vi "FindhInPlane.vi"(3 "Full h(r,t)":bool, 4 "Variables in":T1={"Number of rings"=1, "sound spd (cm/s)"=150000, "z span (cm)"=4.0, "z steps"=20, "y span (cm)"=50.0, "y steps"=0, "time step (s)"=1e-08, "z"=0.0, "y"=0.0, "ref delay"=0.0, "freq (MHz)"=4.71, "cycles"=300} {"freq (MHz)" format="%.2f"; "z span (cm)" format="%.2f"; "y" format="%.2f"; "ref delay" format="%.2f"; "y span (cm)" format="%.2f"; "z" format="%.2f"; "time step (s)" format="%.2e"}, 5 "Trans Geometry":cluster{"Radius":dbl, "a":dbl}={"Radius"=4.8, "a"=1.0} {"a" format="%.2f"; "Radius" format="%.2f"}) -> (0 "Y axis":dbl[](array[numeric]) format="%.2f", 1 "h(r,t)":dbl[][](array[numeric]) format="%.2f", 2 "delay pts":i32[](array[numeric]))   [LabVIEW 2022 SP3]
uses:
  <vilib>/Math Plots/3D Math Plots/3D Surface/3D Surface XCtrl/3D Surface.xctl
  <vilib>/Math Plots/3D Math Plots/3D Surface/3D Surface Datatype/Public/Plot Helper (Matrix).vi
  <vilib>/Math Plots/3D Math Plots/3D Surface/3D Surface Datatype/3D Surface Datatype.lvclass
panel:
  out "3D Surface":refnum<class "3D Plot Datatype.lvclass">[](xcontrol)
  in  "Display 3-D?":bool
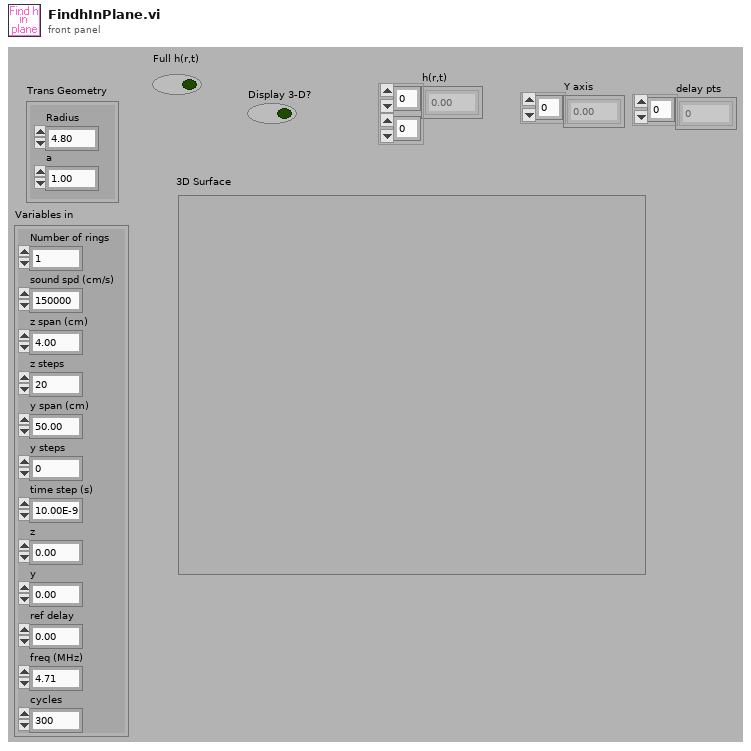
[diagram p1: front panel]
types:
  T1 = cluster{"Number of rings":i32, "sound spd (cm/s)":i32, "z span (cm)":dbl, "z steps":i32, "y span (cm)":dbl, "y steps":i32, "time step (s)":sgl, "z":dbl, "y":dbl, "ref delay":dbl, "freq (MHz)":dbl, "cycles":i32}
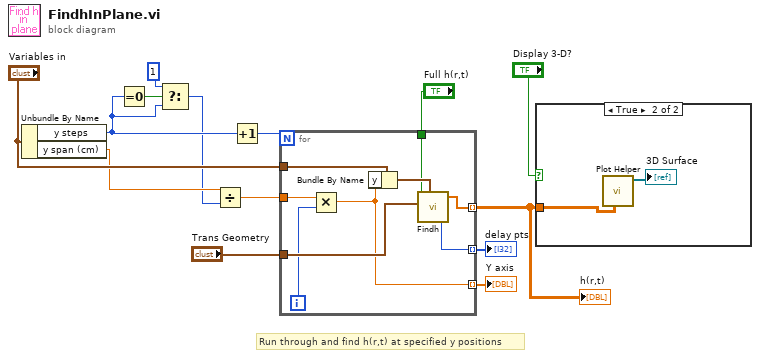
[diagram p0: block diagram]
diagram:
  # "Run through and find h(r,t) at specified y positions"
  n1 = Unbundle By Name("Variables in") -> ("y steps"=w3:i32, "y span (cm)"=w9:dbl)
  n2 = Equal To 0?(x=w3) -> (x = 0?=w4:bool)
  n3 = Select(t=1, s=w4, f=w3) -> (s? t:f=w2:i32)
  n4 = Divide(x=w9, y=w2) -> (x/y=w8:dbl)
  n5 = Increment(x=w3) -> (x+1=w7:i32)
  n6 = for {
    N: w7 -> [_]
    tunnel: "Trans Geometry" -> [w23]
    tunnel: w8 -> [w21]
    tunnel: [w20] -> w14 mode=indexing
    tunnel: "Variables in" -> [w19]
    tunnel: [w18] -> w12 mode=indexing
    tunnel: [w16] -> w6 mode=indexing
    tunnel: "Full h(r,t)" -> [w15]
    i -> [w22]
    n7 = Multiply(x=w21, y=w22) -> (x*y=w18:dbl)
    n8 = Bundle By Name(cluster=w19, "y"=w18) -> (w17:T1)
    n9 = call "Findh.vi"("Full h(r,t)"=w15, "Trans Geometry"=w23, "Variables in"=w17) -> ("h(r,t)"=w20:dbl[], "delay pts"=w16:i32)  [unwired: 3 out]
  }
  "h(r,t)" <- w14
  "Y axis" <- w12
  "delay pts" <- w6
  n10 = case shown="True" "Display 3-D?" {
    tunnel: w14 -> [_ w24]
    frame False {
    }
    frame True {
      n11 = call-poly <vilib>:"Plot Helper.vi"("z matrix"=w24) -> ("3D Plot lvclass Array out"=→"3D Surface":refnum<class "3D Plot Datatype.lvclass">[])  [unwired: 5 in, 5 out]
    }
  }
